vi "Read RPTID File.vi"(8 "error in":errorcluster) -> (0 "error out":errorcluster, 3 "RPTID Data":T1[](array[typedef]))   [LabVIEW 2020, in "SECS Communication.lvlib" / "SECS Data Class.lvclass"]
uses:
  SECS Data Class.lvclass
  RPTID Data.ctl
  <vilib>/DATA AHEAD/XLR8/functions/Workbook/Open Create Workbook XLSX.vi
  <vilib>/DATA AHEAD/XLR8/XLR8.lvlib
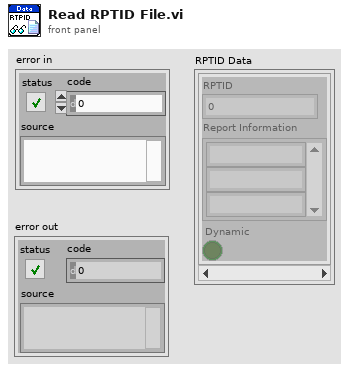
[diagram p1: front panel]
types:
  T1 = typedef "SECS Communication.lvlib/SECS Data Class.lvclass/RPTID Data.ctl" = cluster{"RPTID":u32, "Report Information":string[], "Dynamic":bool}
  T2 = typedef "XLR8.lvlib/XLR8_Ref.ctl" = cluster{"WBK":refnum<k24>, "CurSheet":refnum<k24>, "File":refnum<k24>, "file path":string, "sheet":string, "Sheets":refnum<k24>[], "IsXML":bool, "Policy":i32}
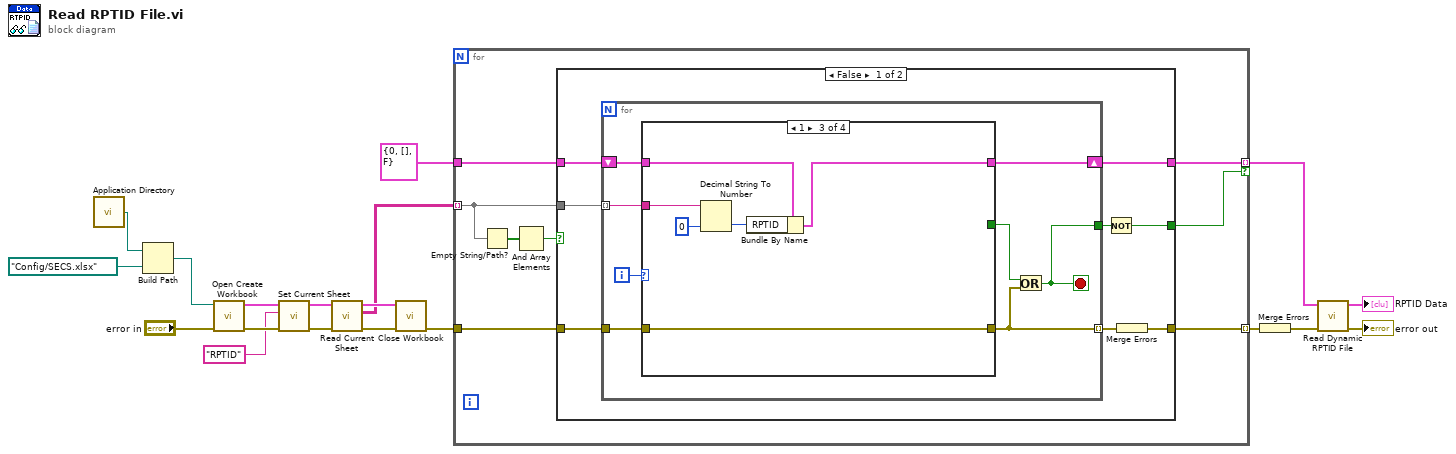
[diagram p0: block diagram]
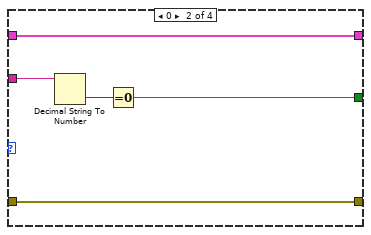
[diagram p3: hidden frame]
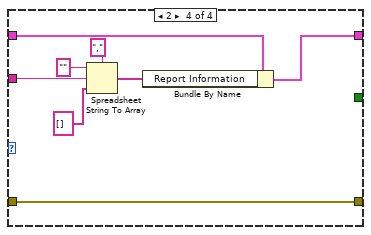
[diagram p4: hidden frame]
diagram:
  n1 = call <vilib>:"Application Directory.vi"() -> ("Application Directory"=w19:path)
  n2 = Build Path(base path=w19, name or relative path=path "Config/SECS.xlsx") -> (appended path=w16:path)
  n3 = call-poly <vilib>:"Open Create Workbook.vi"("error in"="error in", "Workbook Path"=w16) -> ("error out"=w14:errorcluster, "Refs Out"=w15:T2)  [unwired: 8 in]
  n4 = call <vilib>:"Set Current Sheet.vi"("error in"=w14, "Sheet to switch to"="RPTID", "Refs In"=w15) -> ("error out"=w11:errorcluster, "Refs Out"=w12:T2)  [unwired: 7 in]
  n5 = call <vilib>:"Read Current Sheet.vi"("error in"=w11, "Refs In"=w12) -> ("error out"=w9:errorcluster, "Sheet-data out"=w7:string[][], "Refs Out"=w10:T2)  [unwired: 7 in]
  n6 = call <vilib>:"Close Workbook.vi"("error in"=w9, "Refs In"=w10) -> ("error out"=w8:errorcluster)  [unwired: 8 in, 1 out]
  n7 = for {
    tunnel: w8 -> [w24]
    tunnel: w7 -> [w25] mode=indexing
    tunnel: T1 {"RPTID"=0, "Report Information"=[], "Dynamic"=FALSE} ("RPTID Data") -> [w23]
    tunnel: [w22] -> w3 mode=indexing if=w21
    tunnel: [w20] -> w6 mode=indexing
    n8 = Empty String/Path?(string/path=w25) -> (empty?=w27:bool[])
    n9 = And Array Elements(Boolean array=w27) -> (logical AND=w26:bool)
    n10 = case shown="False" w26 {
      tunnel: w25 -> [w35 _]
      tunnel: w24 -> [w30 w65]
      tunnel: w23 -> [w34 w66]
      tunnel: [w33 w66] -> w22
      tunnel: [w31 _] -> w21
      tunnel: [w28 w65] -> w20
      frame False {
        n11 = for {
          tunnel: w35 -> [w41] mode=indexing
          shift-right: [w40] -> w33
          shift-left: w34 -> [w43]
          tunnel: [w36] -> w32
          tunnel: w30 -> [w39]
          tunnel: [w37] -> w29 mode=indexing
          i -> [w42]
          stop <- w36 stop-if-true
          n12 = case shown="1" w42 {
            tunnel: w43 -> [w45 w50 w56 w64]
            tunnel: w41 -> [_ w49 w55 w61]
            tunnel: [w45 w50 w52 w63] -> w40
            tunnel: [_ w47 _ _] -> w38
            tunnel: w39 -> [w44 w46 w51 w62]
            tunnel: [w44 w46 w51 w62] -> w37
            frame Default {
            }
            frame 0 {
              n13 = Decimal String To Number(string=w49) -> (number=w48:i32)  [unwired: 2 in, 1 out]
              n14 = Equal To 0?(x=w48) -> (x = 0?=w47:bool)
            }
            frame 1 {
              n15 = Decimal String To Number(string=w55, default (0L)=u32 0 ("default (0 I32)")) -> (number=w54:u32)  [unwired: 1 in, 1 out]
              n16 = Bundle By Name(cluster=w56, "RPTID"=w54) -> (w52:T1)
            }
            frame 2 {
              n17 = Spreadsheet String To Array(delimiter (Tab)=",", format string="", spreadsheet string=w61, array type (2D Dbl)=string[] []) -> (array=w58:string[])
              n18 = Bundle By Name(cluster=w64, "Report Information"=w58) -> (w63:T1)
            }
          }
          n19 = Or(x=w38, y=w37) -> (x .or. y?=w36:bool)
        }
        n20 = Not(x=w32) -> (.not. x?=w31:bool)
        n21 = Merge Errors(w29) -> (w28:errorcluster)
      }
      frame True {
      }
    }
  }
  n22 = Merge Errors(w6) -> (w4:errorcluster)
  n23 = call "Read Dynamic RPTID File.vi"("error in (no error)"=w4, "RPTID Data In"=w3) -> ("error out"=→"error out":errorcluster, "RPTID Data Out"=→"RPTID Data":T1[])  [unwired: 8 in]
